vi "Load RFP Data FilesPLL.vi"(6 "File Index":i32, 7 "Current Row Number":i32, 8 "Template":path, 9 "Filetype In":string[](array[string]), 10 "File Types to Read":T1, 11 "Files":path[](array[path])) -> (0 "Filetype Out":string[](array[string]), 1 "Channel Values Out":string[][](array[string]), 3 "Ch names Out":string[](array[string]), 4 "File Index Out":i32)   [LabVIEW 2022 SP3]
uses:
  Anemometry/Anemometry Sub Vis/Data_plotting_vis/Data_File_Type.ctl
  Anemometry/Anemometry Sub Vis/Data_plotting_vis/Results_plotter_Global.vi
  Anemometry/Anemometry Sub Vis/Globals/ParallelExecutionGlobal.vi
panel:
  out "nLoadStrands":i32
  out "No Of files":i32
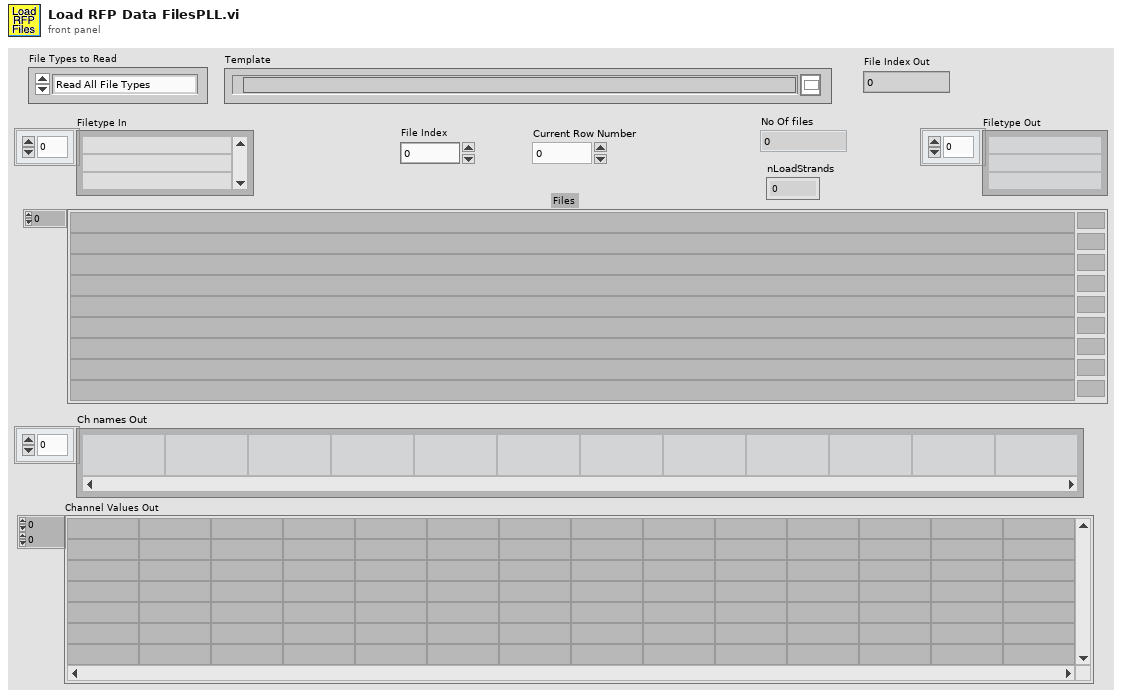
[diagram p1: front panel]
types:
  T1 = typedef "Data_File_Type.ctl" = enum16{"Read All File Types", "Results Files Only", "Raw Data Files Only", "Calibration Files Only", "Gas Desk Files Only", "Old Results Files Only", "Tabulated Data Files Only"}
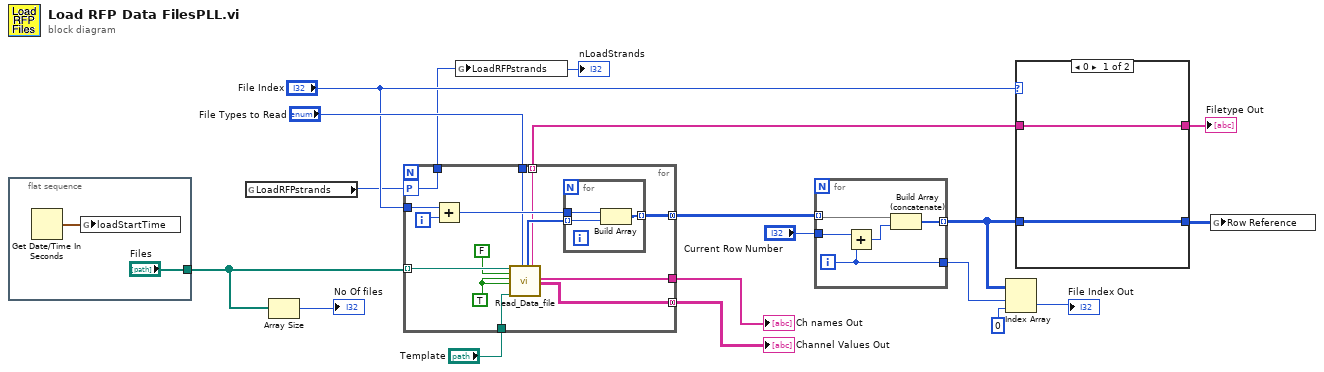
[diagram p0: block diagram]
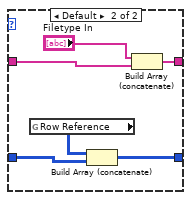
[diagram p2: hidden frame]
diagram:
  n1 = flat-sequence {
    tunnel: ["Files"] -> w4
    frame #0 {
      n2 = Get Date/Time In Seconds() -> (seconds since 1Jan1904=w20:timestamp)
      n3 = global write "Results_plotter_Global.vi" "loadStartTime"(w20) -> ()
    }
  }
  n4 = global read "ParallelExecutionGlobal.vi" "LoadRFPstrands"() -> (w2:i32)
  n5 = Array Size(array=w4) -> (size(s)=→"No Of files":i32)
  n6 = for {
    tunnel: "Template" -> [w34]
    tunnel: w4 -> [w33] mode=indexing
    tunnel: [w31] -> w16 mode=concatenating
    tunnel: [w30] -> w17
    tunnel: "File Index" -> [w28]
    tunnel: [w25] -> w14 mode=concatenating
    tunnel: [w24] -> w15 mode=indexing
    tunnel: "File Types to Read" -> [w23]
    workers-P: w2 -> [w21]
    tunnel: [w21] -> w1
    i -> [w29]
    w22 = TRUE ("Delete First Rows?")
    n7 = Add(x=w28, y=w29) -> (x+y=w27:i32)
    n8 = call "Read_Data_file.vi"("Results file"=w33, "Read Channel Names only"=FALSE, "Delete First Rows?"=w22, "Add Extra Channels?"=w22, "Template File"=w34, "Desired File Types"=w23) -> ("Row numbers"=w26:i32[], "Filetype"=w24:string, "Ch names Out"=w30:string[], "Channel Values Out"=w31:string[][])  [unwired: 1 in, 9 out]
    n9 = for {
      tunnel: w27 -> [w37]
      tunnel: [w36] -> w25 mode=indexing
      tunnel: w26 -> [w35] mode=indexing
      n10 = Build Array(w37, w35) -> (w36:i32[])
    }
  }
  "Channel Values Out" <- w16
  "Ch names Out" <- w17
  "nLoadStrands" <- w1
  n11 = global write "ParallelExecutionGlobal.vi" "LoadRFPstrands"(w1) -> ()
  n12 = for {
    tunnel: w14 -> [w41] mode=indexing
    tunnel: "Current Row Number" -> [w42]
    tunnel: [w39] -> w11 mode=indexing
    tunnel: [w38] -> w10
    i -> [w38]
    n13 = Add(x=w42, y=w38) -> (x+y=w40:i32)
    n14 = Build Array (concatenate)(w41, w40) -> (w39:i32[])
  }
  n15 = Index Array(array=w11, index (row)=w10, index (col)=0 ("disabled index (col)")) -> (element=→"File Index Out":i32)
  n16 = case shown="0" "File Index" {
    tunnel: [w44 w50] -> w12
    tunnel: w11 -> [w44 w49]
    tunnel: w15 -> [w43 w46]
    tunnel: [w43 w45] -> w7
    frame 0 {
    }
    frame Default {
      n17 = global read "Results_plotter_Global.vi" "Row Reference"() -> (w48:i32[][])
      n18 = Build Array (concatenate)(w48, w49) -> (w50:i32[][])
      n19 = Build Array (concatenate)("Filetype In", w46) -> (w45:string[])
    }
  }
  "Filetype Out" <- w7
  n20 = global write "Results_plotter_Global.vi" "Row Reference"(w12) -> ()
